vi "getStopMechClassPath.vi"(5 "stopMechanismType":T1) -> (3 "ITaskClassPath":path)   [LabVIEW 2023]
uses:
  stopMechanismType.ctl
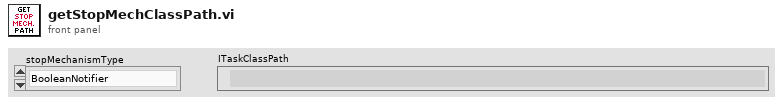
[diagram p1: front panel]
types:
  T1 = typedef "stopMechanismType.ctl" = enum16{"BooleanNotifier", "BooleanUE", "MsgUE"}
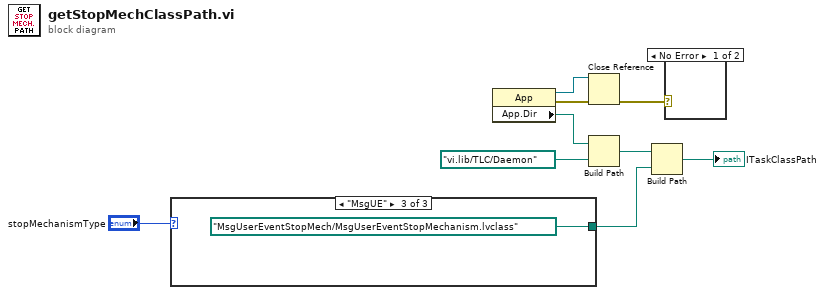
[diagram p0: block diagram]
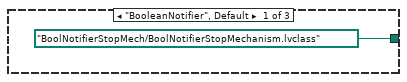
[diagram p3: hidden frame]
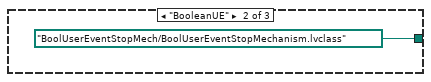
[diagram p4: hidden frame]
diagram:
  n1 = case shown="\"MsgUE\"" "stopMechanismType" {
    tunnel: [path "BoolNotifierStopMech/BoolNotifierStopMechanism.lvclass" ("name or relative path") path "BoolUserEventStopMech/BoolUserEventStopMechanism.lvclass" ("name or relative path") path "MsgUserEventStopMech/MsgUserEventStopMechanism.lvclass" ("name or relative path")] -> w4
    frame "BooleanNotifier", Default {
    }
    frame "BooleanUE" {
    }
    frame "MsgUE" {
    }
  }
  n2 = property class="App"() -> (reference out=w8:refnum<vi>, error out=w9:errorcluster, "App.Dir"=w7:path)  [unwired: 2 in]
  n3 = Close Reference(reference=w8, error in (no error)=w9) -> (error out=w1:errorcluster)
  n4 = Build Path(base path=w7, name or relative path=path "vi.lib/TLC/Daemon") -> (appended path=w3:path)
  n5 = Build Path(base path=w3, name or relative path=w4) -> (appended path=→"ITaskClassPath":path)
  n6 = case shown="No Error" w1 {
    frame No Error {
    }
    frame Error {
    }
  }
